vi "Acquire DAQmx Driver Semaphore.vi"() -> (0 "Semaphore Reference":T1)   [LabVIEW 2013]
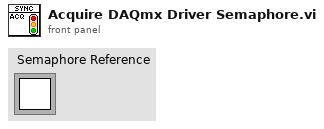
[diagram p1: front panel]
types:
  T1 = typedef "Semaphore RefNum" = refnum<k1>
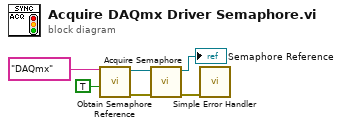
[diagram p0: block diagram]
diagram:
  n1 = call <vilib>:"Obtain Semaphore Reference.vi"("create if not found (T)"=TRUE, "name (unnamed)"="DAQmx") -> ("error out"=w6:errorcluster, "semaphore"=w5:T1)  [unwired: 3 in, 1 out]
  n2 = call <vilib>:"Acquire Semaphore.vi"("error in (no error)"=w6, "semaphore"=w5) -> ("error out"=w1:errorcluster, "semaphore out"=→"Semaphore Reference":T1)  [unwired: 3 in, 1 out]
  n3 = call <vilib>:"Simple Error Handler.vi"("error in (no error)"=w1) -> ()  [unwired: 4 in, 5 out]
